vi "Arduino Tone.vi"() -> ()   [LabVIEW 2011, in "LabVIEW Interface for Arduino.lvlib"]
doc: "An example that uses the arduino's digital output pins to generate a tone that can be played on a speaker or piezo buzzer."
uses:
  vi.lib/LabVIEW Interface for Arduino/LabVIEW Interface for Arduino.lvlib
panel:
  in  "VISA resource name":refnum<visa-resource-name>
  in  "Stop":bool
  in  "Duration ms":u32=1
  in  "Frequency":u16=500 step=100
  in  "Tone DO Pin":u8=8
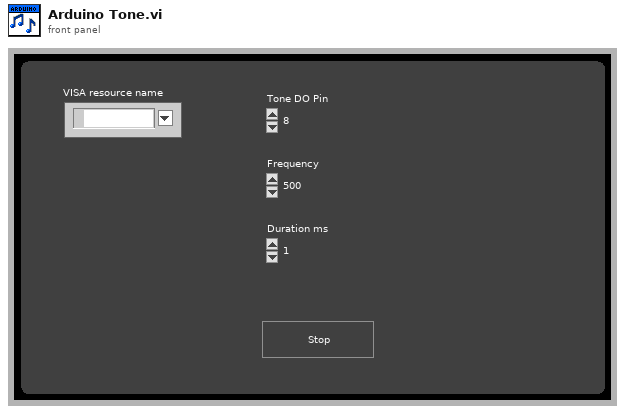
[diagram p1: front panel]
types:
  T1 = typedef "LabVIEW Interface for Arduino.lvlib/Arduino Resource.ctl" = cluster{"VISA resource":refnum<visa-resource-name>, "Board Type":T2, "Connection Type":enum8{"USB / Serial"}, "Bytes Per Packet (15)":u8}
  T2 = typedef "LabVIEW Interface for Arduino.lvlib/Board Type.ctl" = enum16{"Arduino Uno", "Dimuelanove w/Atmega 328", "Mega 2560", "Chipkit Uno32", "Chipkit Max32"}
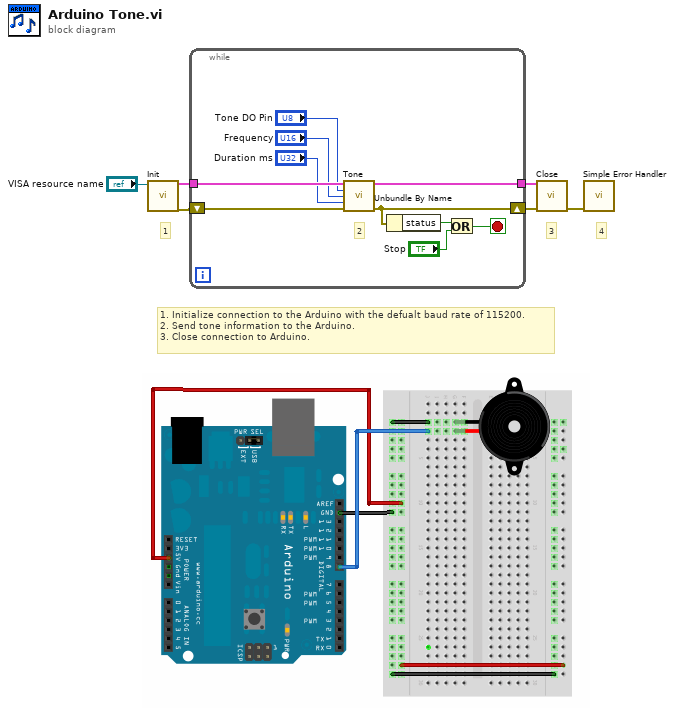
[diagram p0: block diagram]
diagram:
  # "1. Initialize connection to the Arduino with the defualt baud rate of 115200.\n2. Send tone information to the Arduino.\n3. Close connection to Arduino."
  # "4"
  # "3"
  # "1"
  n1 = call "Init.vi"("VISA resource"="VISA resource name") -> ("Arduino Resource"=w6:T1, "error out"=w5:errorcluster)  [unwired: 17 in]
  n2 = while {
    tunnel: w6 -> [w14]
    shift-right: [w11] -> w4
    shift-left: w5 -> [w13]
    tunnel: [w12] -> w3
    stop <- w16 stop-if-true
    # "2"
    n3 = call "Tone.vi"("Arduino Resource"=w14, "Tone DO Pin"="Tone DO Pin", "Frequency (0 Hz)"="Frequency", "Duration (1 ms)"="Duration ms", "error in"=w13) -> ("Arduino Resource"=w12:T1, "error out"=w11:errorcluster)  [unwired: 9 in]
    n4 = Unbundle By Name(w11) -> ("status"=w15:bool)
    n5 = Or(x=w15, y="Stop") -> (x .or. y?=w16:bool)
  }
  n6 = call "Close.vi"("Arduino Resource"=w3, "error in"=w4) -> ("error out"=w2:errorcluster)  [unwired: 13 in]
  n7 = call <vilib>:"Simple Error Handler.vi"("error in (no error)"=w2) -> ()  [unwired: 4 in, 5 out]
